vi "dscCounterRead.vi"(8 "error in":errorcluster, 11 "board":i16) -> (0 "error out":errorcluster, 2 "dsccrOut":T1, 3 "boardOut":i16)   [LabVIEW 2011, in "Diamond Universal Driver.lvlib"]
doc: "Use this template to build a dll driven application for the universal driver on Diamond PC/104 boards. This template sets up the VI for proper error handling and an entry point for the board. However, the <B>Call Library Function</B> node is not configured properly and must be configured by the user."
uses:
  Diamond Universal Driver.lvlib
  Controls/dsccr.ctl
  Controls/dsccs.ctl
  Controls/error codes.ctl
  Instruments/WL OPC/Support/dlls/dscud.dll
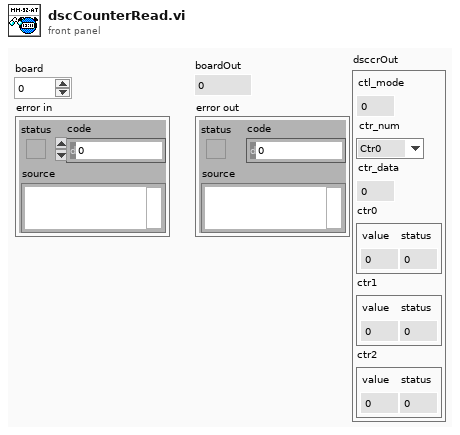
[diagram p1: front panel]
types:
  T1 = typedef "Diamond Universal Driver.lvlib/dsccr.ctl" = cluster{"ctl_mode":u8, "ctr_num":enum8{"Ctr0", "Ctr1", "Ctr2"}, "ctr_data":u32, "ctr0":T2, "ctr1":T2, "ctr2":T2}
  T2 = typedef "Diamond Universal Driver.lvlib/dsccs.ctl" = cluster{"value":u32, "status":u8}
  T3 = typedef "Diamond Universal Driver.lvlib/error codes.ctl" = enum8{"DE_NONE", "DE_HW_FAILURE", "DE_SW_FAILURE", "DE_HW_NOT_SUPPORTED", "DE_SW_NOT_SUPPORTED", "DE_INVALID_PARM", "DE_ALTERNATE_IN_PROGRESS", "DE_NONE_IN_PROGRESS", "DE_BUFFER_ROLLOVER", "DE_INVALID_ERROR_CODE", "DE_ALREADY_PAUSED", "DE_OVERFLOW", "DE_INVALID_FUNC", "DE_DSCUDH_INVALID", "DE_INVALID_BOARD", "DE_BOARD_LIMIT_REACHED", "DE_BOARD_BUSY", "DE_INVALID_WINDRVR_HANDLE", "DE_INVALID_WINDRVR_VERSION", "DE_BAD_WINDRVR_BOARD_INIT", "DE_OPERATION_TIMED_OUT", "DE_INVALID_WINDRVR_KP", "DE_THREAD_FAILURE"}
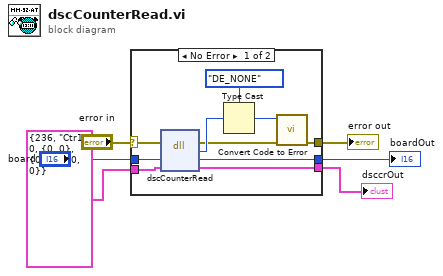
[diagram p0: block diagram]
diagram:
  n1 = case shown="No Error" "error in" {
    selector: "error in" -> [w16 w19]
    tunnel: [w12 w19] -> w5
    tunnel: [w10 w18] -> w4
    tunnel: "board" -> [w9 w18]
    tunnel: T1 {"ctl_mode"=236, "ctr_num"=enum."Ctr1", "ctr_data"=0, "ctr0"={"value"=0, "status"=0}, "ctr1"={"value"=0, "status"=0}, "ctr2"={"value"=0, "status"=0}} ("dsccrIn") -> [w8 w17]
    tunnel: [w7 w17] -> w1
    frame No Error {
      n2 = dll-call lib="C:/Users/mrichardson/Documents/Web Based Version Control SW/Instruments/WL OPC/Support/dlls/dscud.dll" fn="dscCounterRead"(error in=w16, "board"=w9, "dsccr"=w8) -> (error out=w11:errorcluster, "error"=w15:u8, "board"=w10:i16, "dsccr"=w7:T1)  [unwired: 2 in, 1 out]
      n3 = Type Cast(type=error_codes."DE_NONE" ("error codes"), x=w15) -> (*(type *) &x=w13:T3)
      n4 = call "Convert Code to Error.vi"("error in"=w11, "error codes"=w13) -> ("error out"=w12:errorcluster)  [unwired: 9 in]
    }
    frame Error {
    }
  }
  "error out" <- w5
  "boardOut" <- w4
  "dsccrOut" <- w1
